vi "String Tuning High E.vi"(8 "Upper Limit":dbl, 9 "Lower Limit":dbl, 11 "Input Cluster":T1={"Tuner"={"Sharp"=FALSE, "Sharp"=FALSE, "Tuned"=FALSE, "Flat"=FALSE, "Flat"=FALSE}, "Chord"={"A"=FALSE, "B"=FALSE, "C"=FALSE, "D"=FALSE, "E"=FALSE, "F 2"=FALSE, "G"=FALSE}, "Note"={"Low E"=FALSE, "A"=FALSE, "D"=FALSE, "G"=FALSE, "B"=FALSE, "High E"=FALSE}, "Frequency Spectrum 2"=[{"t0"=timestamp(3721854148.349081 s since 1904-01-01), "dt"=0.0003333, "Y"=array[1000 elements], "attributes"=variant("NI_ChannelName"=variant(string "Voltage"), "NI_UnitDescription"=variant(string "Volts"))}]}) -> (1 "Tuned":bool, 3 "Output Cluster":T1={"Tuner"={"Sharp"=FALSE, "Sharp"=FALSE, "Tuned"=FALSE, "Flat"=FALSE, "Flat"=FALSE}, "Chord"={"A"=FALSE, "B"=FALSE, "C"=FALSE, "D"=FALSE, "E"=FALSE, "F 2"=FALSE, "G"=FALSE}, "Note"={"Low E"=FALSE, "A"=FALSE, "D"=FALSE, "G"=FALSE, "B"=FALSE, "High E"=FALSE}, "Frequency Spectrum 2"=[{"t0"=timestamp(3721854148.349081 s since 1904-01-01), "dt"=0.0003333, "Y"=array[1000 elements], "attributes"=variant("NI_ChannelName"=variant(string "Voltage"), "NI_UnitDescription"=variant(string "Volts"))}]})   [LabVIEW 2020]
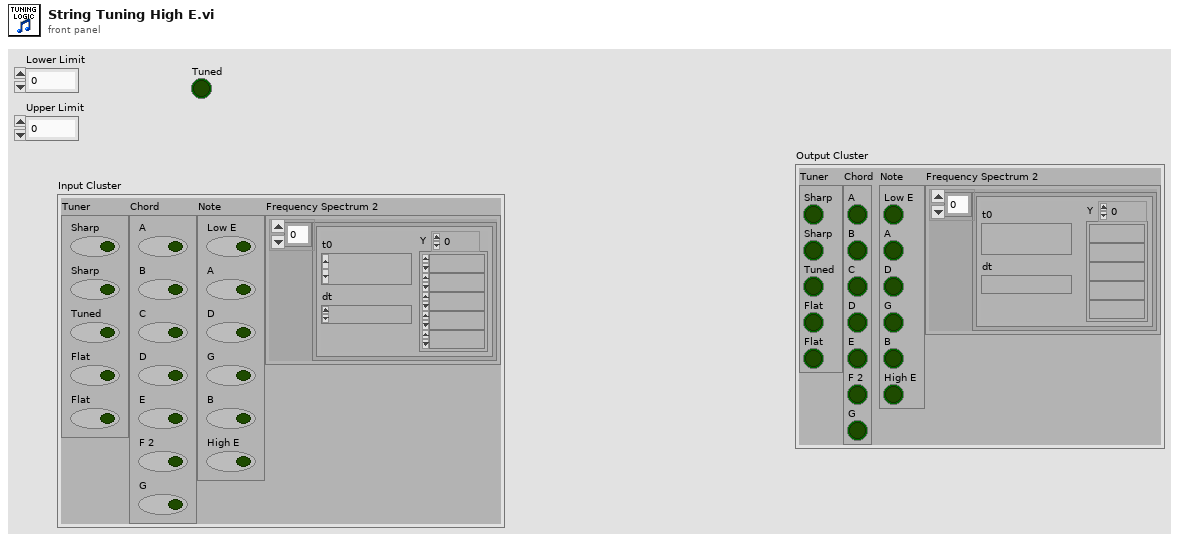
[diagram p1: front panel]
types:
  T1 = cluster{"Tuner":cluster{"Sharp":bool, "Sharp":bool, "Tuned":bool, "Flat":bool, "Flat":bool}, "Chord":cluster{"A":bool, "B":bool, "C":bool, "D":bool, "E":bool, "F 2":bool, "G":bool}, "Note":cluster{"Low E":bool, "A":bool, "D":bool, "G":bool, "B":bool, "High E":bool}, "Frequency Spectrum 2":dynamicdata}
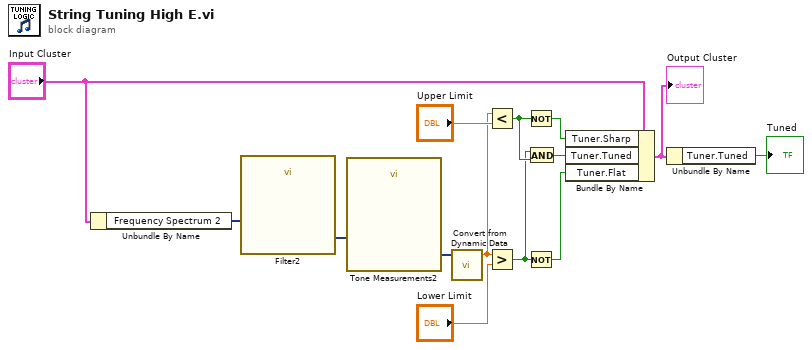
[diagram p0: block diagram]
diagram:
  n1 = Unbundle By Name("Input Cluster") -> ("Frequency Spectrum 2"=w3:dynamicdata)
  n2 = call "Filter2"("Signal"=w3) -> ("Filtered Signal"=w2:dynamicdata)  [unwired: 9 in, 1 out]
  n3 = call "Tone Measurements2"("Signals"=w2) -> ("Frequency"=w1:dynamicdata)  [unwired: 9 in, 1 out]
  n4 = call "Convert from Dynamic Data"("Dynamic Data Type"=w1) -> ("Scalar"=w7:dbl)  [unwired: 3 in]
  n5 = Less?(x=w7, y="Upper Limit") -> (x < y?=w13:bool)
  n6 = Greater?(x=w7, y="Lower Limit") -> (0:w11:bool)
  n7 = Not(x=w13) -> (.not. x?=w14:bool)
  n8 = Not(x=w11) -> (.not. x?=w12:bool)
  n9 = And(x=w11, y=w13) -> (x .and. y?=w10:bool)
  n10 = Bundle By Name(cluster="Input Cluster", "Tuner.Sharp"=w14, "Tuner.Tuned"=w10, "Tuner.Flat"=w12) -> (w4:T1)
  "Output Cluster" <- w4
  n11 = Unbundle By Name(w4) -> ("Tuner.Tuned"=→"Tuned":bool)
